vi "Excel_Read_Array.vi"(4 "Cell Range 2":string="C2", 6 "Cell Range 1":string="C2", 7 "Worksheet Number":i32=1, 8 "error in (no error)":errorcluster, 9 "Sheets Reference In":refnum<k7>) -> (0 "error out":errorcluster, 1 "Sheets Reference Out":refnum<k7>, 2 "Read Values Array":dbl[][](array[numeric]))   [LabVIEW 2014]
doc: "This VI demonstrates the use of ActiveX to write a table into a Microsoft Excel worksheet."
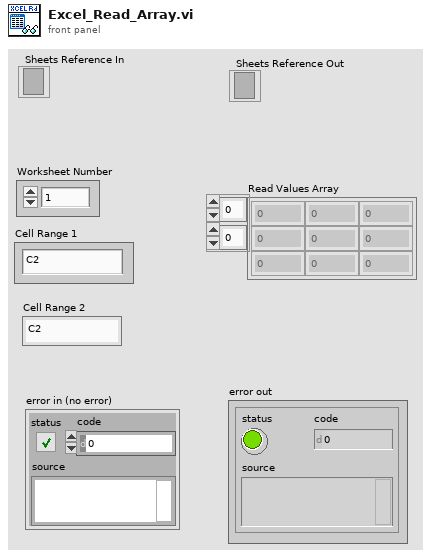
[diagram p1: front panel]
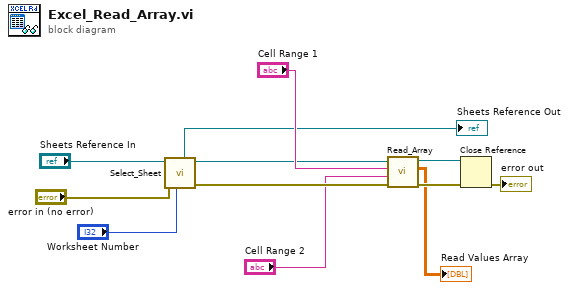
[diagram p0: block diagram]
diagram:
  n1 = call "Select_Sheet.vi"("Worksheet Number"="Worksheet Number", "error in (no error)"="error in (no error)", "Automation Refnum in"="Sheets Reference In") -> ("error out"=w5:errorcluster, "Automation Refnum out"=w6:refnum<k7>, "Sheets Refnum"=→"Sheets Reference Out":refnum<k7>)  [unwired: 6 in]
  n2 = call "Read_Array.vi"("error in (no error)"=w5, "Range 2 to Read"="Cell Range 2", "Range 1 to Read"="Cell Range 1", "Automation Refnum in"=w6) -> ("error out"=w9:errorcluster, "Read Values Array"=→"Read Values Array":dbl[][], "reference out"=w10:refnum<k7>)  [unwired: 5 in]
  n3 = Close Reference(reference=w10, error in (no error)=w9) -> (error out=→"error out":errorcluster)
